vi "Swerve Steer Configs.vi"(1 "Max Encoder Val":dbl=360.0, 2 "Input IDs":T1, 3 "PID Constants":T2={"P Gain"=0.0, "I Gain"=0.0, "D Gain"=0.0, "F Gain"=0.0, "I Zone"=0.0, "Min Output"=-1.0, "Max Output"=1.0}) -> ()   [LabVIEW 2023]
doc: "A quick bundle to initialize all Swerve Steer motors. \nFUTURE NOTE: Consider adding individual PID controls based on performance."
uses:
  <vilib>/Rock Robotics/WPI/ThirdParty/REV Robotics/REVLib/Typedef/Spark MAX Sensor Type.ctl
  <vilib>/Rock Robotics/WPI/ThirdParty/REV Robotics/REVLib/Typedef/Spark MAX Idle Mode.ctl
  <vilib>/Rock Robotics/WPI/ThirdParty/REV Robotics/REVLib/Typedef/Spark MAX Motor Type.ctl
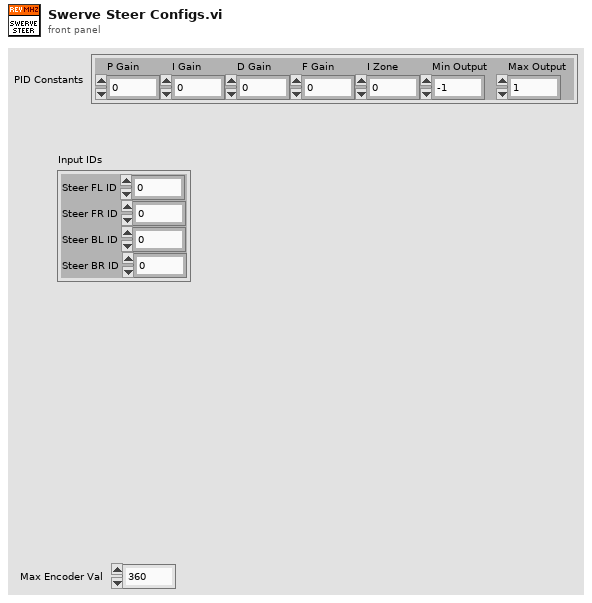
[diagram p1: front panel]
types:
  T1 = cluster{"Steer FL ID":u8, "Steer FR ID":u8, "Steer BL ID":u8, "Steer BR ID":u8}
  T2 = cluster{"P Gain":dbl, "I Gain":dbl, "D Gain":dbl, "F Gain":dbl, "I Zone":dbl, "Min Output":dbl, "Max Output":dbl}
  T3 = typedef "Spark MAX Motor Type.ctl" = enum16{"Brushed", "Brushless"}
  T4 = typedef "Spark MAX Idle Mode.ctl" = enum16{"Coast", "Brake"}
  T5 = typedef "Spark MAX Sensor Type.ctl" = enum16{"No Sensor", "Hall Sensor", "Encoder", "-Not Available-", "Analog", "Alternate Encoder", "Duty Cycle"}
  T6 = typedef "WPI_MotorControlDeviceRef.ctl" = cluster{"DeviceStatus":errorcluster, "Type":T7, "PWM":cluster{"PWM Channel":T8, "DeadBand":T9}, "CAN":cluster{"Device Number":u8, "SetOutput VI Ref":variant, "GetOutput VI Ref":variant, "Enable VI Ref":variant, "Disable VI Ref":variant, "Data":variant}, "Invert":bool, "DIO PWM":cluster{"PWM \"Enable\" Channel":T8, "DIOChannel":T10, "PWM Rate":dbl}}
  T7 = typedef "WPI_MotorControlType.ctl" = enum16{"PWM", "CAN", "DIO PWM"}
  T8 = typedef "FPGA_DIOPWMChannel.ctl" = enum8{"PWM 0", "PWM 1", "PWM 2", "PWM 3", "PWM 4", "PWM 5", "PWM 6", "PWM 7", "PWM 8", "PWM 9", "PWM MXP 0", "PWM MXP 1", "PWM MXP 2", "PWM MXP 3", "PWM MXP 4", "PWM MXP 5", "PWM MXP 6", "PWM MXP 7", "PWM MXP 8", "PWM MXP 9", "Invalid"}
  T9 = typedef "WPI_PWMDeadband.ctl" = cluster{"Name":string, "maxPositivePwm":i32, "minPositivePwm":i32, "centerPwm":i32, "maxNegativePwm":i32, "minNegativePwm":i32, "angularRange":u16}
  T10 = typedef "FPGA_DIOChannel.ctl" = enum8{"DIO 0", "DIO 1", "DIO 2", "DIO 3", "DIO 4", "DIO 5", "DIO 6", "DIO 7", "DIO 8", "DIO 9", "DIO MXP 0", "DIO MXP 1", "DIO MXP 2", "DIO MXP 3", "DIO MXP 4", "DIO MXP 5", "DIO MXP 6", "DIO MXP 7", "DIO MXP 8", "DIO MXP 9", "DIO MXP 10", "DIO MXP 11", "DIO MXP 12", "DIO MXP 13", "DIO MXP 14", "DIO MXP 15", "SPI Port CS1", "SPI Port CS2", "SPI Port CS3", "SPI Port MISO", "SPI Port MOSI", "Invalid"}
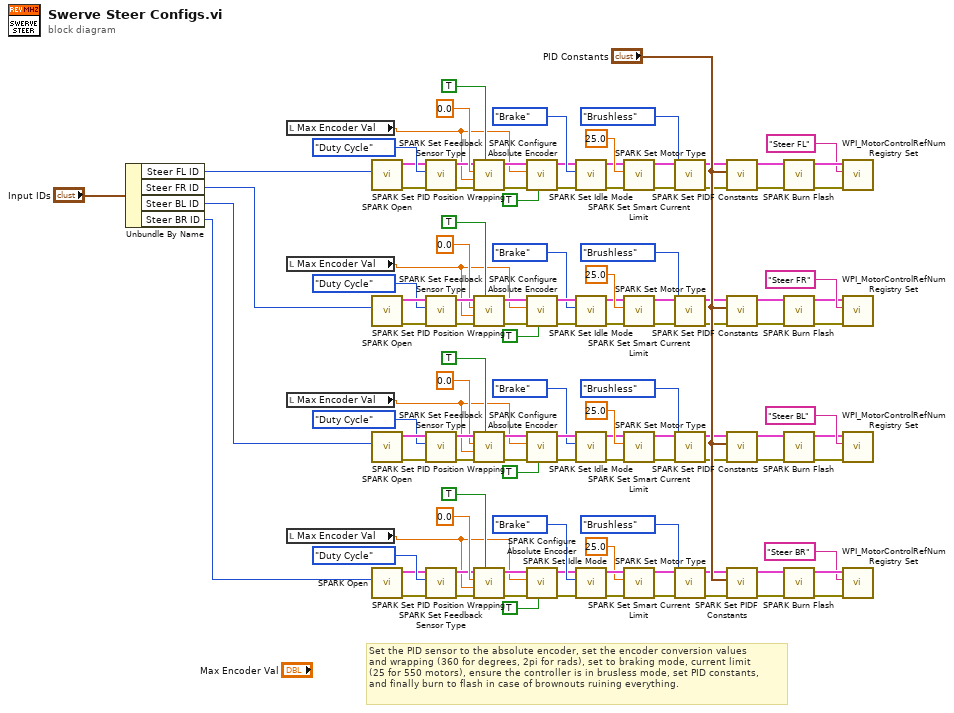
[diagram p0: block diagram]
diagram:
  # "Set the PID sensor to the absolute encoder, set the encoder conversion values\nand wrapping (360 for degrees, 2pi for rads), set to braking mode, current limit\n(25 for 550 motors), ensure the controller is in brusless mode, set PID constants,\nand finally burn to flash in case of brownouts ruining everything."
  n1 = Unbundle By Name("Input IDs") -> ("Steer FL ID"=w4:u8, "Steer FR ID"=w3:u8, "Steer BL ID"=w2:u8, "Steer BR ID"=w1:u8)
  n2 = local read "Max Encoder Val"() -> (w42:dbl)
  n3 = local read "Max Encoder Val"() -> (w41:dbl)
  n4 = local read "Max Encoder Val"() -> (w40:dbl)
  n5 = local read "Max Encoder Val"() -> (w39:dbl)
  n6 = call <vilib>:"SPARK Open.vi"("Device Number"=w4) -> ("error out"=w102:errorcluster, "MotorControlDeviceRef"=w104:T6)  [unwired: 9 in]
  n7 = call <vilib>:"SPARK Open.vi"("Device Number"=w3) -> ("error out"=w95:errorcluster, "MotorControlDeviceRef"=w93:T6)  [unwired: 9 in]
  n8 = call <vilib>:"SPARK Open.vi"("Device Number"=w2) -> ("error out"=w63:errorcluster, "MotorControlDeviceRef"=w61:T6)  [unwired: 9 in]
  n9 = call <vilib>:"SPARK Open.vi"("Device Number"=w1) -> ("error out"=w70:errorcluster, "MotorControlDeviceRef"=w72:T6)  [unwired: 9 in]
  n10 = call <vilib>:"SPARK Set Feedback Sensor Type.vi"("error in (no error)"=w102, "Sensor Type"=Spark_MAX_Sensor_Type."Duty Cycle", "MotorControlDevRef"=w104) -> ("error out"=w103:errorcluster, "MotorControlDeviceRef"=w105:T6)  [unwired: 7 in]
  n11 = call <vilib>:"SPARK Set Feedback Sensor Type.vi"("error in (no error)"=w95, "Sensor Type"=Spark_MAX_Sensor_Type."Duty Cycle", "MotorControlDevRef"=w93) -> ("error out"=w94:errorcluster, "MotorControlDeviceRef"=w92:T6)  [unwired: 7 in]
  n12 = call <vilib>:"SPARK Set Feedback Sensor Type.vi"("error in (no error)"=w63, "Sensor Type"=Spark_MAX_Sensor_Type."Duty Cycle", "MotorControlDevRef"=w61) -> ("error out"=w62:errorcluster, "MotorControlDeviceRef"=w60:T6)  [unwired: 7 in]
  n13 = call <vilib>:"SPARK Set Feedback Sensor Type.vi"("error in (no error)"=w70, "Sensor Type"=Spark_MAX_Sensor_Type."Duty Cycle", "MotorControlDevRef"=w72) -> ("error out"=w71:errorcluster, "MotorControlDeviceRef"=w73:T6)  [unwired: 7 in]
  n14 = call <vilib>:"SPARK Set PID Position Wrapping.vi"("Enable (F)"=TRUE, "error in (no error)"=w103, "Maximum Output (0)"=w42, "Minimum Input (0)"=0.0, "MotorControlDeviceRef in"=w105) -> ("error out"=w108:errorcluster, "MotorControlDeviceRef out"=w109:T6)  [unwired: 5 in]
  n15 = call <vilib>:"SPARK Set PID Position Wrapping.vi"("Enable (F)"=TRUE, "error in (no error)"=w94, "Maximum Output (0)"=w41, "Minimum Input (0)"=0.0, "MotorControlDeviceRef in"=w92) -> ("error out"=w89:errorcluster, "MotorControlDeviceRef out"=w88:T6)  [unwired: 5 in]
  n16 = call <vilib>:"SPARK Set PID Position Wrapping.vi"("Enable (F)"=TRUE, "error in (no error)"=w62, "Maximum Output (0)"=w40, "Minimum Input (0)"=0.0, "MotorControlDeviceRef in"=w60) -> ("error out"=w57:errorcluster, "MotorControlDeviceRef out"=w56:T6)  [unwired: 5 in]
  n17 = call <vilib>:"SPARK Set PID Position Wrapping.vi"("Enable (F)"=TRUE, "error in (no error)"=w71, "Maximum Output (0)"=w39, "Minimum Input (0)"=0.0, "MotorControlDeviceRef in"=w73) -> ("error out"=w76:errorcluster, "MotorControlDeviceRef out"=w77:T6)  [unwired: 5 in]
  n18 = call <vilib>:"SPARK Configure Absolute Encoder.vi"("Inverted (F)"=TRUE, "error in (no error)"=w108, "Position Conversion Factor (1)"=w42, "MotorControlDeviceRef in"=w109) -> ("error out"=w112:errorcluster, "MotorControlDeviceRef out"=w113:T6)  [unwired: 6 in]
  n19 = call <vilib>:"SPARK Configure Absolute Encoder.vi"("Inverted (F)"=TRUE, "error in (no error)"=w89, "Position Conversion Factor (1)"=w41, "MotorControlDeviceRef in"=w88) -> ("error out"=w85:errorcluster, "MotorControlDeviceRef out"=w84:T6)  [unwired: 6 in]
  n20 = call <vilib>:"SPARK Configure Absolute Encoder.vi"("Inverted (F)"=TRUE, "error in (no error)"=w57, "Position Conversion Factor (1)"=w40, "MotorControlDeviceRef in"=w56) -> ("error out"=w53:errorcluster, "MotorControlDeviceRef out"=w52:T6)  [unwired: 6 in]
  n21 = call <vilib>:"SPARK Configure Absolute Encoder.vi"("Inverted (F)"=TRUE, "error in (no error)"=w76, "Position Conversion Factor (1)"=w39, "MotorControlDeviceRef in"=w77) -> ("error out"=w80:errorcluster, "MotorControlDeviceRef out"=w81:T6)  [unwired: 6 in]
  n22 = call <vilib>:"SPARK Set Idle Mode.vi"("error in (no error)"=w112, "Idle Mode"=Spark_MAX_Idle_Mode."Brake", "MotorControlDeviceRef in"=w113) -> ("error out"=w12:errorcluster, "MotorControlDeviceRef out"=w13:T6)  [unwired: 7 in]
  n23 = call <vilib>:"SPARK Set Idle Mode.vi"("error in (no error)"=w85, "Idle Mode"=Spark_MAX_Idle_Mode."Brake", "MotorControlDeviceRef in"=w84) -> ("error out"=w10:errorcluster, "MotorControlDeviceRef out"=w11:T6)  [unwired: 7 in]
  n24 = call <vilib>:"SPARK Set Idle Mode.vi"("error in (no error)"=w53, "Idle Mode"=Spark_MAX_Idle_Mode."Brake", "MotorControlDeviceRef in"=w52) -> ("error out"=w24:errorcluster, "MotorControlDeviceRef out"=w22:T6)  [unwired: 7 in]
  n25 = call <vilib>:"SPARK Set Idle Mode.vi"("error in (no error)"=w80, "Idle Mode"=Spark_MAX_Idle_Mode."Brake", "MotorControlDeviceRef in"=w81) -> ("error out"=w37:errorcluster, "MotorControlDeviceRef out"=w36:T6)  [unwired: 7 in]
  n26 = call <vilib>:"SPARK Set Smart Current Limit.vi"("error in (no error)"=w12, "Primay Current Limit (80A)"=25.0, "MotorControlDeviceRef in"=w13) -> ("error out"=w20:errorcluster, "MotorControlDeviceRef out"=w19:T6)  [unwired: 7 in]
  n27 = call <vilib>:"SPARK Set Smart Current Limit.vi"("error in (no error)"=w10, "Primay Current Limit (80A)"=25.0, "MotorControlDeviceRef in"=w11) -> ("error out"=w15:errorcluster, "MotorControlDeviceRef out"=w16:T6)  [unwired: 7 in]
  n28 = call <vilib>:"SPARK Set Smart Current Limit.vi"("error in (no error)"=w24, "Primay Current Limit (80A)"=25.0, "MotorControlDeviceRef in"=w22) -> ("error out"=w27:errorcluster, "MotorControlDeviceRef out"=w28:T6)  [unwired: 7 in]
  n29 = call <vilib>:"SPARK Set Smart Current Limit.vi"("error in (no error)"=w37, "Primay Current Limit (80A)"=25.0, "MotorControlDeviceRef in"=w36) -> ("error out"=w34:errorcluster, "MotorControlDeviceRef out"=w33:T6)  [unwired: 7 in]
  n30 = call <vilib>:"SPARK Set Motor Type.vi"("error in (no error)"=w20, "Motor Type"=Spark_MAX_Motor_Type."Brushless", "MotorControlDevRef"=w19) -> ("error out"=w8:errorcluster, "MotorControlDeviceRef"=w9:T6)  [unwired: 7 in]
  n31 = call <vilib>:"SPARK Set Motor Type.vi"("error in (no error)"=w15, "Motor Type"=Spark_MAX_Motor_Type."Brushless", "MotorControlDevRef"=w16) -> ("error out"=w6:errorcluster, "MotorControlDeviceRef"=w7:T6)  [unwired: 7 in]
  n32 = call <vilib>:"SPARK Set Motor Type.vi"("error in (no error)"=w27, "Motor Type"=Spark_MAX_Motor_Type."Brushless", "MotorControlDevRef"=w28) -> ("error out"=w25:errorcluster, "MotorControlDeviceRef"=w23:T6)  [unwired: 7 in]
  n33 = call <vilib>:"SPARK Set Motor Type.vi"("error in (no error)"=w34, "Motor Type"=Spark_MAX_Motor_Type."Brushless", "MotorControlDevRef"=w33) -> ("error out"=w31:errorcluster, "MotorControlDeviceRef"=w32:T6)  [unwired: 7 in]
  n34 = call <vilib>:"SPARK Set PIDF Constants.vi"("error in"=w8, "PID Constants"="PID Constants", "MotorControlDeviceRef"=w9) -> ("error out"=w49:errorcluster, "MotorControlDeviceRef"=w50:T6)  [unwired: 7 in]
  n35 = call <vilib>:"SPARK Set PIDF Constants.vi"("error in"=w6, "PID Constants"="PID Constants", "MotorControlDeviceRef"=w7) -> ("error out"=w44:errorcluster, "MotorControlDeviceRef"=w43:T6)  [unwired: 7 in]
  n36 = call <vilib>:"SPARK Set PIDF Constants.vi"("error in"=w25, "PID Constants"="PID Constants", "MotorControlDeviceRef"=w23) -> ("error out"=w46:errorcluster, "MotorControlDeviceRef"=w45:T6)  [unwired: 7 in]
  n37 = call <vilib>:"SPARK Set PIDF Constants.vi"("error in"=w31, "PID Constants"="PID Constants", "MotorControlDeviceRef"=w32) -> ("error out"=w47:errorcluster, "MotorControlDeviceRef"=w48:T6)  [unwired: 7 in]
  n38 = call <vilib>:"SPARK Burn Flash.vi"("error in"=w49, "MotorControlDeviceRef"=w50) -> ("error out"=w101:errorcluster, "MotorControlDeviceRef"=w100:T6)  [unwired: 8 in]
  n39 = call <vilib>:"SPARK Burn Flash.vi"("error in"=w44, "MotorControlDeviceRef"=w43) -> ("error out"=w96:errorcluster, "MotorControlDeviceRef"=w97:T6)  [unwired: 8 in]
  n40 = call <vilib>:"SPARK Burn Flash.vi"("error in"=w46, "MotorControlDeviceRef"=w45) -> ("error out"=w64:errorcluster, "MotorControlDeviceRef"=w65:T6)  [unwired: 8 in]
  n41 = call <vilib>:"SPARK Burn Flash.vi"("error in"=w47, "MotorControlDeviceRef"=w48) -> ("error out"=w69:errorcluster, "MotorControlDeviceRef"=w68:T6)  [unwired: 8 in]
  n42 = call <vilib>:"WPI_MotorControlRefNum Registry Set.vi"("error in (no error)"=w101, "refnum name"="Steer FL" ("Change to match from begin.vi"), "MotorControlDevRef"=w100) -> ()  [unwired: 7 in, 2 out]
  n43 = call <vilib>:"WPI_MotorControlRefNum Registry Set.vi"("error in (no error)"=w96, "refnum name"="Steer FR" ("Change to match from begin.vi"), "MotorControlDevRef"=w97) -> ()  [unwired: 7 in, 2 out]
  n44 = call <vilib>:"WPI_MotorControlRefNum Registry Set.vi"("error in (no error)"=w64, "refnum name"="Steer BL" ("Change to match from begin.vi"), "MotorControlDevRef"=w65) -> ()  [unwired: 7 in, 2 out]
  n45 = call <vilib>:"WPI_MotorControlRefNum Registry Set.vi"("error in (no error)"=w69, "refnum name"="Steer BR" ("Change to match from begin.vi"), "MotorControlDevRef"=w68) -> ()  [unwired: 7 in, 2 out]
